vi "Randomize Colors.vi"(0 "Next Sample Start Position":i32, 1 "Cycle Colors?":bool, 2 "Iteration":i32, 5 "Current Max":dbl, 7 "Levels":dbl[](graph)=[0.72967529296875, 0.57769775390625, 0.634521484375, 0.887969970703125, 0.760345458984375, 0.63958740234375, 0.4696044921875, 0.87945556640625, 0.782501220703125, 0.600006103515625, 0.382080078125, 0.405029296875, 0.890869140625, 0.6834716796875, 0.530609130859375, 0.429473876953125, 0.599151611328125, 0.46832275390625, 0.50018310546875, 0.396575927734375, 0.757080078125, 0.720550537109375, 0.69842529296875, 0.524749755859375, 0.63189697265625, 0.63922119140625, 0.78045654296875, 0.537017822265625, 0.8701171875, 0.7677001953125, 0.63916015625, 0.40191650390625, 0.566162109375], 9 "Threshold Multilier":dbl=1.0, 11 "error in":errorcluster) -> (4 "Next Sample Start Position":i32, 8 "Levels":dbl[](graph)=[0.72967529296875, 0.57769775390625, 0.634521484375, 0.887969970703125, 0.760345458984375, 0.63958740234375, 0.4696044921875, 0.87945556640625, 0.782501220703125, 0.600006103515625, 0.382080078125, 0.405029296875, 0.890869140625, 0.6834716796875, 0.530609130859375, 0.429473876953125, 0.599151611328125, 0.46832275390625, 0.50018310546875, 0.396575927734375, 0.757080078125, 0.720550537109375, 0.69842529296875, 0.524749755859375, 0.63189697265625, 0.63922119140625, 0.78045654296875, 0.537017822265625, 0.8701171875, 0.7677001953125, 0.63916015625, 0.40191650390625, 0.566162109375], 10 "Color":u32(colorbox), 15 "error out":errorcluster)   [LabVIEW 2015, in "LabVIEW Interface for Arduino.lvlib"]
uses:
  <vilib>/LabVIEW Interface for Arduino/LabVIEW Interface for Arduino.lvlib
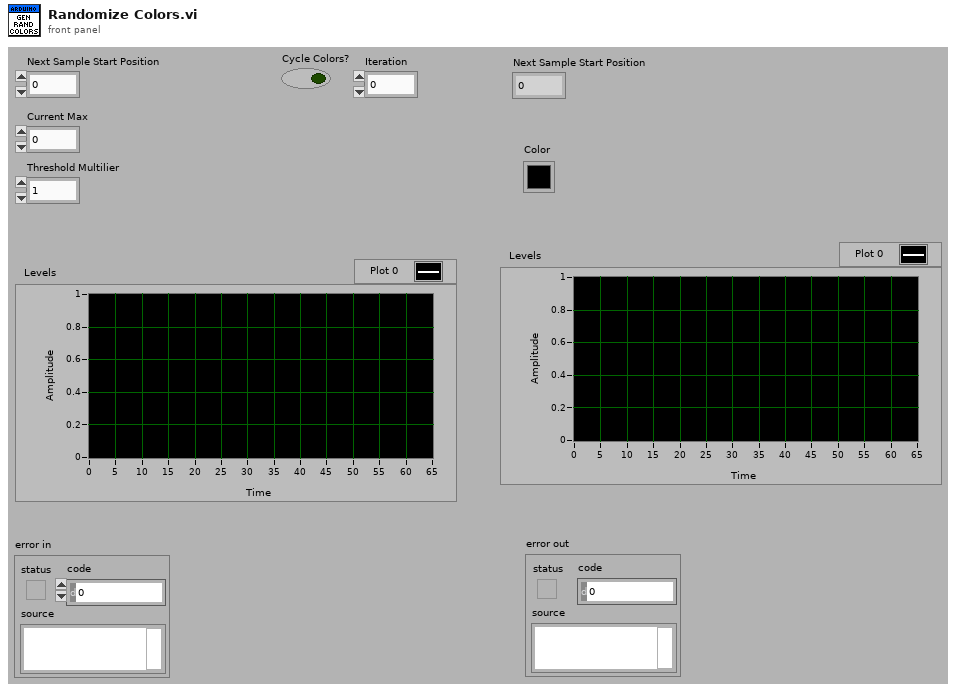
[diagram p1: front panel]
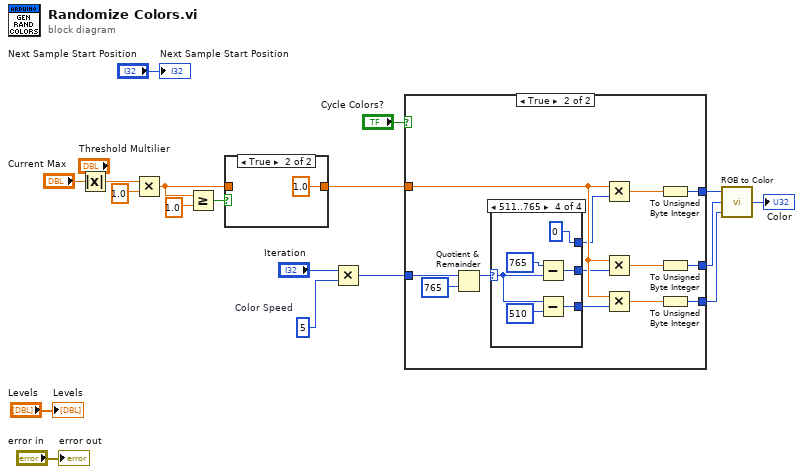
[diagram p0: block diagram]
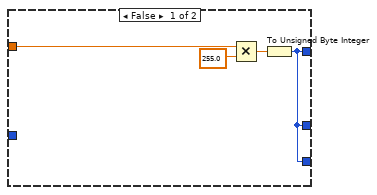
[diagram p2: hidden frame]
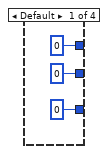
[diagram p3: hidden frame]
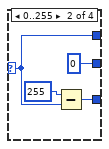
[diagram p4: hidden frame]
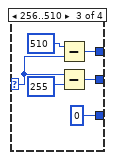
[diagram p5: hidden frame]
diagram:
  w15 = 5  # Color Speed
  n1 = Absolute Value(x="Current Max") -> (abs(x)=w9:dbl)
  n2 = Multiply(x=w9, y=1.0) -> (x*y=w13:dbl)
  n3 = Greater Or Equal?(x=w13, y=1.0) -> (x >= y?=w12:bool)
  n4 = case shown="True" w12 {
    tunnel: w13 -> [w19 _]
    tunnel: [w19 1.0 ("y")] -> w14
    frame False {
    }
    frame True {
    }
  }
  n5 = Multiply(x="Iteration", y=w15) -> (x*y=w17:i32)
  n6 = case shown="True" "Cycle Colors?" {
    tunnel: w17 -> [_ w35]
    tunnel: w14 -> [w22 w34]
    tunnel: [w24 w27] -> w6
    tunnel: [w24 w26] -> w7
    tunnel: [w24 w25] -> w8
    frame False {
      n7 = Multiply(x=w22, y=255.0) -> (x*y=w21:dbl)
      n8 = To Unsigned Byte Integer(number=w21) -> (unsigned 8bit integer=w24:u8)
    }
    frame True {
      n9 = Quotient & Remainder(x=w35, y=765) -> (x-y*floor(x/y)=w37:i32)  [unwired: 1 out]
      n10 = case shown="511..765" w37 {
        selector: w37 -> [_ w44 w45 w52]
        tunnel: [0 ("y") w44 w48 0 ("y")] -> w33
        tunnel: [0 0 w49 w53] -> w32
        tunnel: [0 ("y") w42 u8 0 ("y") w54] -> w31
        frame Default {
        }
        frame 0..255 {
          n11 = Subtract(x=255, y=w44) -> (x-y=w42:i32)
        }
        frame 256..510 {
          n12 = Subtract(x=510 ("y"), y=w45) -> (x-y=w48:i32)
          n13 = Subtract(x=w45, y=255) -> (x-y=w49:i32)
        }
        frame 511..765 {
          n14 = Subtract(x=765, y=w52) -> (x-y=w53:i32)
          n15 = Subtract(x=w52, y=510) -> (x-y=w54:i32)
        }
      }
      n16 = Multiply(x=w34, y=w33) -> (x*y=w30:dbl)
      n17 = Multiply(x=w34, y=w32) -> (x*y=w29:dbl)
      n18 = Multiply(x=w34, y=w31) -> (x*y=w28:dbl)
      n19 = To Unsigned Byte Integer(number=w30) -> (unsigned 8bit integer=w25:u8)
      n20 = To Unsigned Byte Integer(number=w29) -> (unsigned 8bit integer=w26:u8)
      n21 = To Unsigned Byte Integer(number=w28) -> (unsigned 8bit integer=w27:u8)
    }
  }
  n22 = call <vilib>:"RGB to Color.vi"("B"=w6, "G"=w7, "R"=w8) -> ("Color"=→"Color":u32)
  "Next Sample Start Position" <- "Next Sample Start Position"
  "error out" <- "error in"
  "Levels" <- "Levels"
